vi "artInitParm.vi"() -> (0 "初始化参数":dbl[](array[numeric]))   [LabVIEW 2018]
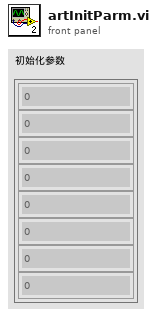
[diagram p1: front panel]
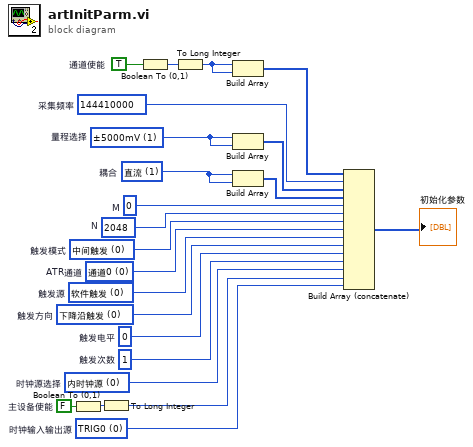
[diagram p0: block diagram]
diagram:
  w6 = 2048  # N
  w7 = 0  # M
  w8 = 1 items=["交流", "直流"]  # 耦合
  w4 = 1 items=["±1000mV", "±5000mV"]  # 量程选择
  w10 = TRUE  # 通道使能
  w2 = 144410000  # 采集频率
  w13 = 0 items=["中间触发", "后触发", "预触发", "硬件延时触发"]  # 触发模式
  w11 = 0 items=["通道0", "通道1"]  # ATR通道
  w21 = 0 items=["软件触发", "DTR作为触发源", "ATR作为触发源", "Trigger信号触发"]  # 触发源
  w20 = 0 items=["下降沿触发", "上升沿触发", "上下边沿均触发", ""]  # 触发方向
  w19 = 0  # 触发电平
  w5 = 1  # 触发次数
  w17 = 0 items=["TRIG0", "TRIG1", "TRIG2", "TRIG3"]  # 时钟输入输出源
  w23 = FALSE  # 主设备使能
  w18 = 0 items=["内时钟源", "主卡10M时钟源", "外部时钟"]  # 时钟源选择
  n1 = Boolean To (0,1) ("布尔值至(0,1)转换")(Boolean=w23) -> (0, 1=w15:i16)
  n2 = To Long Integer(number=w15) -> (32bit integer=w16:i32)
  n3 = Boolean To (0,1)(Boolean=w10) -> (0, 1=w14:i16)
  n4 = To Long Integer(number=w14) -> (32bit integer=w9:i32)
  n5 = Build Array(w9, w9) -> (w3:i32[])
  n6 = Build Array(w4, w4) -> (w12:i32[])
  n7 = Build Array(w8, w8) -> (w22:i32[])
  n8 = Build Array (concatenate) ("创建数组")(w3, w2, w12, w22, w7, w6, w13, w11, w21, w20, w19, w5, w18, w16, w17) -> (→"初始化参数":i32[])
